vi "Main.vi"() -> ()   [LabVIEW 2018]
doc: "The myRIO Project template acquires acceleration data from the onboard accelerometer and displays the changes of acceleration values in a waveform chart."
uses:
  <vilib>/myRIO/Common/Instrument Driver Framework/myRIO v1.0/UART/vis/myRIO v1.0 Close UART.vi
  <vilib>/Utility/error.llb/Error Cluster From Error Code.vi
  <vilib>/myRIO/Common/Instrument Driver Framework/myRIO v1.0/PWM/vis/myRIO v1.0 Write PWM.vi
  <vilib>/myRIO/Common/Instrument Driver Framework/myRIO v1.0/AI/vis/myRIO v1.0 Read AI.vi
  <vilib>/myRIO/Common/Instrument Driver Framework/myRIO v1.0/DIO/vis/myRIO v1.0 Read DIO.vi
  <vilib>/myRIO/Common/Instrument Driver Framework/myRIO v1.0/DIO/vis/myRIO v1.0 Write DIO.vi
  <vilib>/myRIO/Common/Instrument Driver Framework/Utilities/vis/FPGA Ref Manager.vi
  <vilib>/myRIO/Common/Instrument Driver Framework/myRIO v1.0/myRIO v1.0 Reset FPGA.vi
  <vilib>/myRIO/Common/Instrument Driver Framework/myRIO v1.0/IRQ/vis/myRIO v1.0 IRQ Info FGV.vi
  <vilib>/myRIO/Common/Instrument Driver Framework/myRIO v1.0/IRQ/vis/myRIO v1.0 Timer IRQ Info FGV.vi
  <vilib>/myRIO/Common/Instrument Driver Framework/myRIO v1.0/IRQ/vis/myRIO v1.0 ISR Agent.vi
  <vilib>/myRIO/Instrument Drivers/Utilities/Utilities.lvlib
  <vilib>/myRIO/Instrument Drivers/Onboard IO/PWM/PWM.lvlib
  <vilib>/myRIO/Instrument Drivers/Onboard IO/AI/AI.lvlib
  <vilib>/myRIO/Instrument Drivers/Onboard IO/DIO/DIO.lvlib
panel:
  in  "Stepper frekvens":dbl=350.0
  out "ALL BOTTOM":bool
  out "ALL TOP":bool
  in  "Test bor (T = Amperestyring)":bool
  in  "DIR":bool
  in  "Endstops":bool
  in  "Manuel stepper?":bool
  in  "Enum":T1(ring)
  out "Batteri tilbage (%)":dbl
  out "Mean 50":dbl format="%0.2f"
  out "Mean 100":dbl format="%0.2f"
  in  "Threshold forskel":dbl=0.02 format="%#_13g"
  out "Duty Cycle":dbl
  in  "Styr manuelt?":bool=TRUE
  out "Waveform Chart":dbl(graph)
  out "Målt ampere":dbl
  in  "Bor - Frequency [Hz]":dbl=200.0
  in  "Bor - Duty Cycle":dbl=50.0
  out "error out":errorcluster
  in  "Stop":bool
  # "WIRING:\nBrun = GND\nOrange = PWM (A/DIO8)"
  # "STYRING AF SYSTEM!"
  # "100 = max\n50 = 0\n0 = -max"
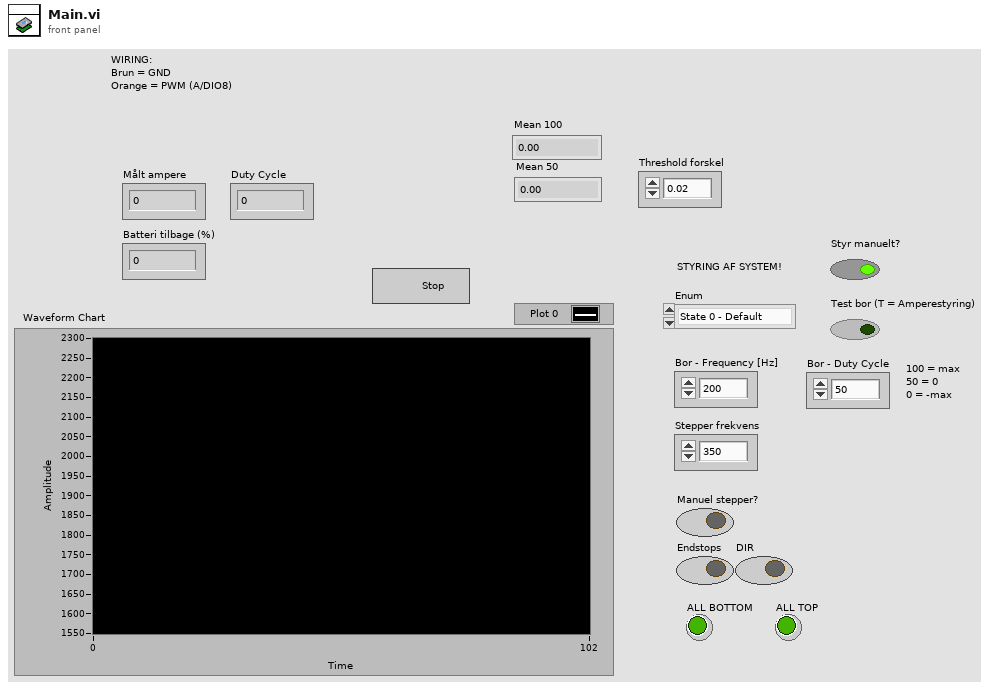
[diagram p1: front panel]
types:
  T1 = enum16{"State 0 - Default", "State 1 - Go down", "State 2 - Go up"}
  T2 = typedef "DIO.lvlib/DIO Reference.ctl" = cluster{"myRIO Reference":T3, "DIO Channels List":T7}
  T3 = typedef "myRIO Generic Hardware Reference.ctl" = cluster{"myRIO Model":T4, "myRIO Hardware Reference":T5}
  T4 = typedef "Hardware Version Enum.ctl" = enum16{"Unknown", "myRIO-1900", "myRIO-1950", "roboRIO", "NI ELVIS RIO CM", "ELVIS III"}
  T5 = typedef "myRIO v1.0 Reference.ctl" = cluster{"Generic FPGA Reference":T6, "Allow multiple opens":bool}
  T6 = typedef "Generic FPGA Reference.ctl" = refnum<k20>
  T7 = typedef "DIO Channels List.ctl" = T8[]
  T8 = typedef "DIO Channels Enum.ctl" = enum16{"Not Connected", "C/DIO0", "C/DIO1", "C/DIO2", "C/DIO3", "C/DIO4", "C/DIO5", "C/DIO6", "C/DIO7", "A/DIO0", "A/DIO1", "A/DIO2", "A/DIO3", "A/DIO4", "A/DIO5", "A/DIO6", "A/DIO7", "A/DIO8", "A/DIO9", "A/DIO10", "A/DIO11", "A/DIO12", "A/DIO13", "A/DIO14", "A/DIO15", "A/DIO16", "A/DIO17", "A/DIO18", "A/DIO19", "B/DIO0", "B/DIO1", "B/DIO2", "B/DIO3", "B/DIO4", "B/DIO5", "B/DIO6", "B/DIO7", "B/DIO8", "B/DIO9", "B/DIO10", "B/DIO11", "B/DIO12", "B/DIO13", "B/DIO14", "B/DIO15", "B/DIO16", "B/DIO17", "B/DIO18", "B/DIO19", "LED0", "LED1", "LED2", "LED3", "Button0", "DIO/DIO0", "DIO/DIO1", "DIO/DIO2", "DIO/DIO3", "DIO/DIO4", "DIO/DIO5", "DIO/DIO6", "DIO/DIO7", "DIO/DIO8", "DIO/DIO9", "SPI/CS0", "SPI/CS1", "SPI/CS2", "SPI/CS3", "LED RADIO (Green)", "LED RADIO (Red)", "LED COMM (Green)", "LED COMM (Red)", "LED MODE (Green)", "LED MODE (Red)"}
  T9 = typedef "PWM.lvlib/PWM Reference.ctl" = cluster{"myRIO Reference":T3, "PWM Channels Enum":T10, "PWM Configuration":T11}
  T10 = typedef "PWM Channels Enum.ctl" = enum16{"Not Connected", "C/PWM0", "C/PWM1", "A/PWM0", "A/PWM1", "A/PWM2", "A/PWM3", "A/PWM4", "A/PWM5", "A/PWM6", "A/PWM7", "A/PWM8", "A/PWM9", "A/PWM10", "A/PWM11", "A/PWM12", "A/PWM13", "A/PWM14", "A/PWM15", "A/PWM16", "A/PWM17", "A/PWM18", "A/PWM19", "B/PWM0", "B/PWM1", "B/PWM2", "B/PWM3", "B/PWM4", "B/PWM5", "B/PWM6", "B/PWM7", "B/PWM8", "B/PWM9", "B/PWM10", "B/PWM11", "B/PWM12", "B/PWM13", "B/PWM14", "B/PWM15", "B/PWM16", "B/PWM17", "B/PWM18", "B/PWM19", "PWM/PWM0", "PWM/PWM1", "PWM/PWM2", "PWM/PWM3", "PWM/PWM4", "PWM/PWM5", "PWM/PWM6", "PWM/PWM7", "PWM/PWM8", "PWM/PWM9"}
  T11 = typedef "PWM.lvlib/PWM Configuration.ctl" = cluster{"Frequency":dbl, "Duty Cycle":dbl}
  T12 = typedef "Accelerometer.lvlib/Accelerometer Reference.ctl" = cluster{"myRIO Reference":T3, "Accelerometer Channels List":T13, "LSB Weight":dbl}
  T13 = typedef "Accelerometer Channels List.ctl" = T14[]
  T14 = typedef "Accelerometer Channels Enum.ctl" = enum16{"Not Connected", "X-Axis", "Y-Axis", "Z-Axis"}
  T15 = typedef "AI.lvlib/AI Reference.ctl" = cluster{"myRIO Reference":T3, "AI Channels List":T16, "AI Scaling Constants List":T18}
  T16 = typedef "AI Channels List.ctl" = T17[]
  T17 = typedef "AI Channels Enum.ctl" = enum16{"Not Connected", "AudioIn/Left", "AudioIn/Right", "C/AI0", "C/AI1", "A/AI0", "A/AI1", "A/AI2", "A/AI3", "A/AI4", "A/AI5", "A/AI6", "A/AI7", "B/AI0", "B/AI1", "B/AI2", "B/AI3", "B/AI4", "B/AI5", "B/AI6", "B/AI7", "AI/AI0", "AI/AI1", "AI/AI2", "AI/AI3", "A/AI0 (DIFF)", "A/AI1 (DIFF)", "A/AI2 (DIFF)", "A/AI3 (DIFF)", "B/AI0 (DIFF)", "B/AI1 (DIFF)", "B/AI2 (DIFF)", "B/AI3 (DIFF)"}
  T18 = typedef "Analog Scaling Constants List.ctl" = T19[]
  T19 = typedef "Analog Scaling Constants.ctl" = cluster{"LSB Weight (Volts)":dbl, "Offset (Volts)":dbl, "Signed?":bool}
  T20 = typedef "SPI.lvlib/SPI Reference.ctl" = cluster{"myRIO Reference":T3, "SPI Channels Enum":T21, "SPI Configuration":T22}
  T21 = typedef "SPI Channels Enum.ctl" = enum16{"Not Connected", "A/SPI", "B/SPI", "SPI/SPI"}
  T22 = typedef "SPI.lvlib/SPI Configuration.ctl" = cluster{"Frequency [Hz]":dbl, "Clock Phase":T23, "Clock Polarity":T24, "Data Direction":T25, "Frame Length":T26}
  T23 = typedef "SPI Clock Phase.ctl" = enum8{"Leading", "Trailing"}
  T24 = typedef "SPI Clock Polarity.ctl" = enum8{"Low", "High"}
  T25 = typedef "SPI Data Direction.ctl" = enum8{"Most significant bit first", "Least significant bit first"}
  T26 = typedef "SPI Frame Length.ctl" = u8
  T27 = cluster{"B/DIO0 - Stepper Direction":T2, "B/DIO1 - Stepper1 Enable":T2, "B/DIO2 - Stepper2 Enable":T2, "B/DIO3 - Stepper3 Enable":T2, "B/DIO4 - Endstop Stepper1 Top":T2, "B/DIO11 - Endstop Stepper1 Bund":T2, "B/DIO12 - Endstop Stepper2 Top":T2, "B/DIO13 - Endstop Stepper2 Bund":T2, "B/DIO14 - Endstop Stepper3 Top":T2, "B/DIO15 - Endstop Stepper3 Bund":T2, "A/DIO0 - Cooler":T2, "A/DIO1 - Beacon drop (dio1)":T2, "A/DIO2 - Beacon drop (dio0)":T2, "A/DIO3 - QuickRelease (dio1)":T2, "A/DIO4 - QuickRelease (dio0)":T2, "A/DIO11 - LiDAR SPI CS":T2, "B/PWM0 - Stepper":T9, "B/PWM1 - Drill":T9, "A/PWM0 - Servo_Roll":T9, "A/PWM1 - Servo_Yaw":T9, "Acc. X-axis":T12, "Acc. Y-axis":T12, "B/AI0 - Drone Grounded F3":T15, "B/AI1 - Drone Drill Gear F4":T15, "B/AI2 - Beacon Drop F5":T15, "B/AI3 - Drone Drill Boost F6":T15, "A/AI0 - Drone Stepper F8":T15, "A/AI1 - Beacon Wiper":T15, "A/AI2 - QuickRelease Wiper":T15, "A/AI3 - Drill Current":T15, "A/SPI - LiDAR":T20, "B/UART - XBee":refnum<visa-resource-name>, "A/UART - A3 GPS":refnum<visa-resource-name>, "RIO Flashing LEDs":T2}
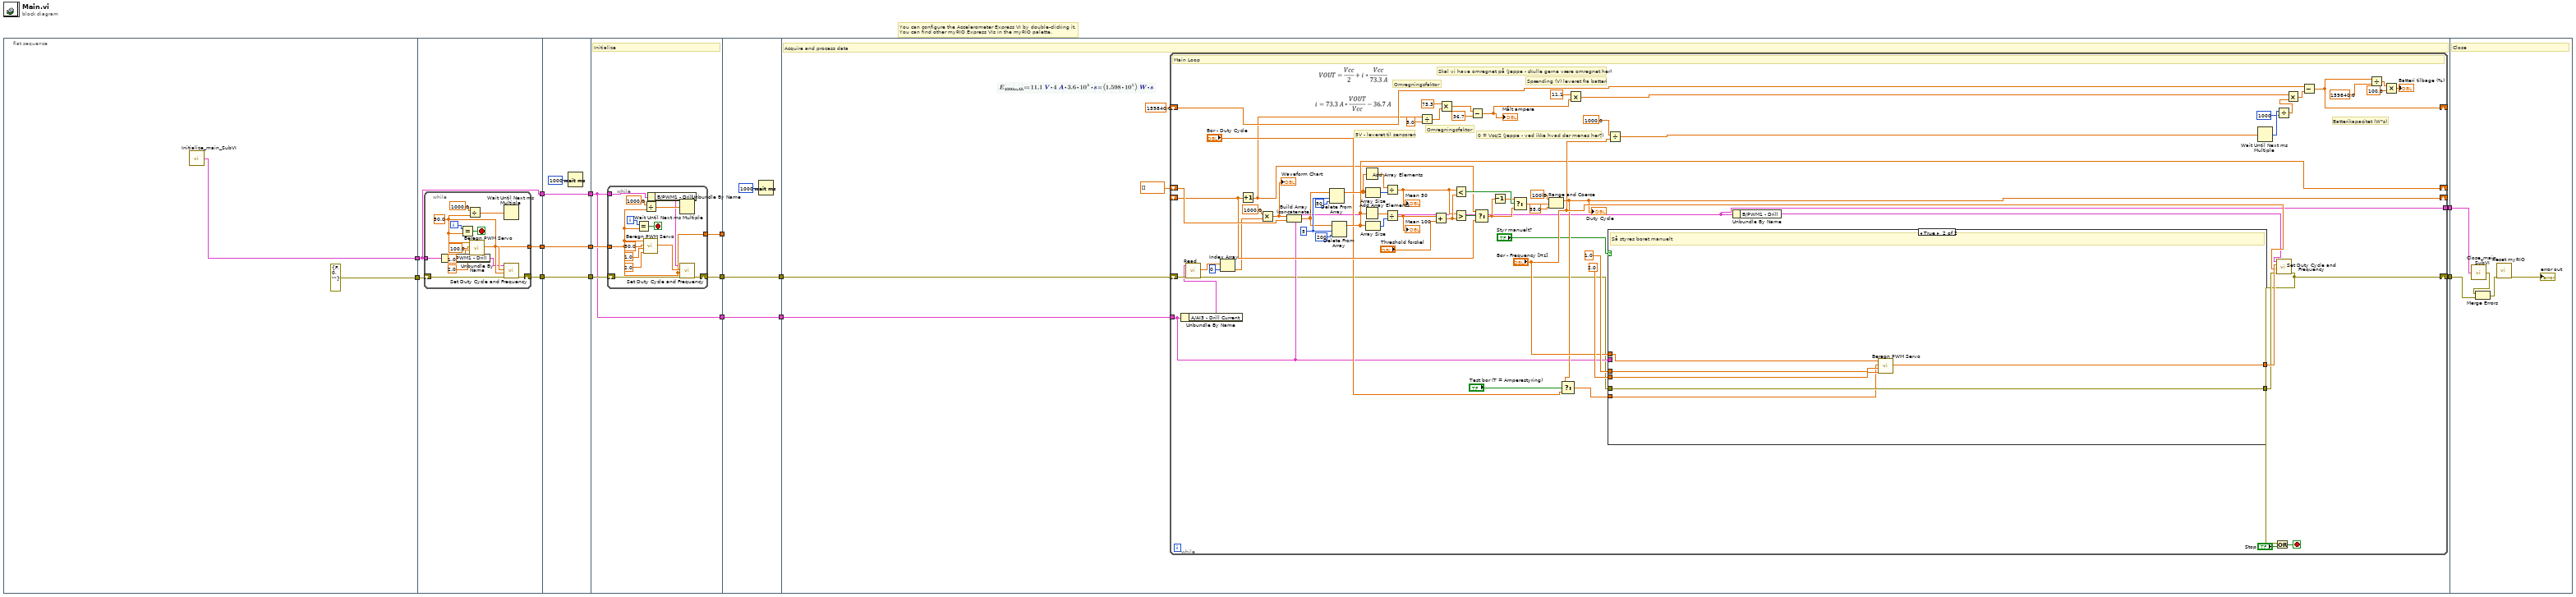
[diagram p0: block diagram]
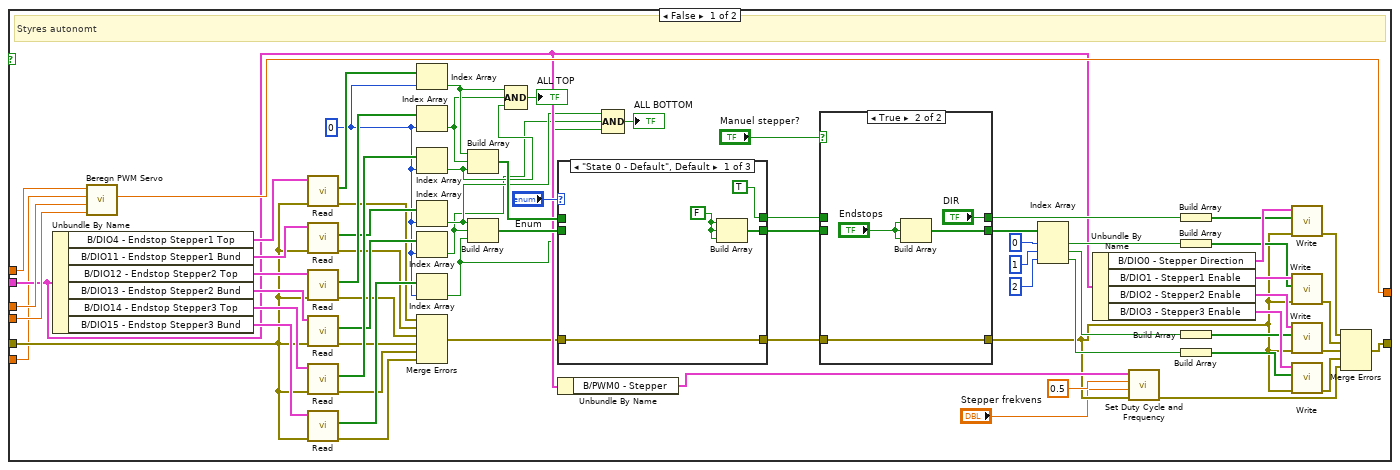
[diagram p2: hidden frame]
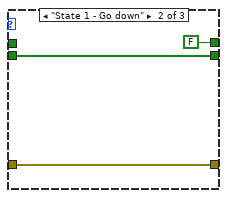
[diagram p4: hidden frame]
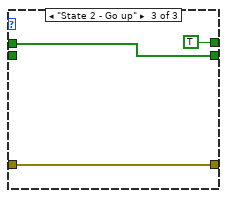
[diagram p5: hidden frame]
diagram:
  # "You can configure the Accelerometer Express VI by double-clicking it.\nYou can find other myRIO Express VIs in the myRIO palette."
  n1 = flat-sequence {
    tunnel: [w17] -> w8
    tunnel: [errorcluster {"status"=FALSE, "code"=0, "source"=""} ("error constant")] -> w2
    tunnel: [w21] -> w13
    tunnel: [w20] -> w11
    tunnel: w8 -> [w19]
    tunnel: [w19] -> w7
    tunnel: w2 -> [w18]
    tunnel: [w37] -> w14
    tunnel: w13 -> [w37]
    tunnel: [w36] -> w12
    tunnel: w11 -> [w36]
    tunnel: w7 -> [w35]
    tunnel: [w35] -> w6
    tunnel: w14 -> [w43]
    tunnel: w12 -> [w42]
    tunnel: [w40] -> w10
    tunnel: [w41] -> w9
    tunnel: w6 -> [w39]
    tunnel: [w39] -> w4
    tunnel: w10 -> [w57]
    tunnel: w9 -> [_]
    tunnel: [w58] -> w5
    tunnel: w4 -> [w58]
    tunnel: [w57] -> w3
    tunnel: [w65] -> w15
    tunnel: w5 -> [w62]
    tunnel: w3 -> [w61]
    tunnel: [w60] -> w1
    tunnel: w15 -> [w226]
    tunnel: w1 -> [w224]
    frame #0 {
      n2 = call "Initialize_main_SubVI.vi"() -> ("output cluster"=w17:T27)
    }
    frame #1 {
      n3 = while {
        tunnel: [w26] -> w21
        shift-right: [w29] -> w20
        shift-left: w18 -> [w30]
        tunnel: w19 -> [w23]
        i -> [w28]
        stop <- w24 stop-if-true
        w26 = 50.0 ("Frequency [Hz]")
        n4 = Unbundle By Name(w23) -> ("B/PWM1 - Drill"=w22:T9)
        n5 = Equal?(x=w28, y=w26) -> (x = y?=w24:bool)
        n6 = Divide(x=1000.0, y=w26) -> (x/y=w27:dbl)
        n7 = call "Beregn PWM Servo.vi"("Max (ms puls bredde)"=2.0, "Min (ms puls bredde)"=1.0, "Duty Cycle"=100.0, "Frekvens"=w26) -> ("Output Dutycycle til PWM Servo"=w31:dbl)  [unwired: 7 in]
        n8 = Wait Until Next ms Multiple(millisecond multiple=w27) -> ()  [unwired: 1 out]
        n9 = call <vilib>:"Set Duty Cycle and Frequency.vi"("error in (no error)"=w30, "Frequency [Hz]"=w26, "Duty Cycle"=w31, "PWM Ref In"=w22) -> ("error out"=w29:errorcluster)  [unwired: 5 in, 1 out]
      }
    }
    frame #2 {
      n10 = Wait (ms)(milliseconds to wait=u32 1000) -> ()  [unwired: 1 out]
    }
    frame #3 {
      # "Initialize"
      n11 = while {
        tunnel: [w46] -> w41
        shift-right: [w51] -> w40
        shift-left: w42 -> [w52]
        tunnel: w43 -> [w46]
        tunnel: w39 -> [w45]
        i -> [w50]
        stop <- w47 stop-if-true
        n12 = Equal?(x=w50, y=w46) -> (x = y?=w47:bool)
        n13 = call "Beregn PWM Servo.vi"("Max (ms puls bredde)"=2.0, "Min (ms puls bredde)"=1.0, "Duty Cycle"=50.0, "Frekvens"=w46) -> ("Output Dutycycle til PWM Servo"=w53:dbl)  [unwired: 7 in]
        n14 = Divide(x=1000.0, y=w46) -> (x/y=w49:dbl)
        n15 = Unbundle By Name(w45) -> ("B/PWM1 - Drill"=w44:T9)
        n16 = Wait Until Next ms Multiple(millisecond multiple=w49) -> ()  [unwired: 1 out]
        n17 = call <vilib>:"Set Duty Cycle and Frequency.vi"("error in (no error)"=w52, "Frequency [Hz]"=w46, "Duty Cycle"=w53, "PWM Ref In"=w44) -> ("error out"=w51:errorcluster)  [unwired: 5 in, 1 out]
      }
    }
    frame #4 {
      n18 = Wait (ms)(milliseconds to wait=u32 1000) -> ()  [unwired: 1 out]
    }
    frame #5 {
      # "Acquire and process data"
      n19 = while {
        shift-right: [w69] -> w65
        shift-left: w61 -> [w118]
        shift-right: [w104] -> _
        shift-left: dbl[] [] -> [w128]
        shift-right: [w77] -> _
        shift-left: _ -> [w125]
        shift-right: [w82] -> _
        shift-left: 159840.0 -> [w83]
        tunnel: w62 -> [w72]
        tunnel: [w72] -> w60
        stop <- w131 stop-if-true
        w111 = 5 ("length")
        # "Batterikapacitet (W*s)"
        # "Spænding (V) leveret fra batteri"
        # "Omregningsfaktor"
        # "Omregningsfaktor"
        # "5V - leveret til sensoren"
        # "Skal vi have omregnet på (Jeppe - skulle gerne være omregnet her)"
        # "0 = Vcc/2 (Jeppe - ved ikke hvad der menes her?)"
        # "Main Loop"
        n20 = Unbundle By Name(w72) -> ("A/AI3 - Drill Current"=w74:T15)
        n21 = call <vilib>:"Read.vi"("error in (no error)"=w118, "AI Ref In"=w74) -> ("error out"=w71:errorcluster, "Values"=w117:dbl[])  [unwired: 7 in, 1 out]
        n22 = Index Array(array=w117, index=0) -> (element=w98:dbl)
        n23 = Increment(x=w125) -> (x+1=w68:dbl)
        n24 = Multiply(x=1000.0, y=w98) -> (x*y=w96:dbl)
        "Waveform Chart" <- w96
        n25 = Build Array (concatenate)(w96, w128) -> (w109:dbl[])
        n26 = Delete From Array(array=w109, length=w111, index=50) -> (array with subset deleted=w100:dbl[])  [unwired: 1 out]
        n27 = Delete From Array(array=w109, length=w111, index=200) -> (array with subset deleted=w104:dbl[])  [unwired: 1 out]
        n28 = Add Array Elements(numeric array=w100) -> (sum=w101:dbl)
        n29 = Add Array Elements(numeric array=w104) -> (sum=w106:dbl)
        n30 = Array Size(array=w100) -> (size(s)=w102:i32)
        n31 = Array Size(array=w104) -> (size(s)=w105:i32)
        n32 = Divide(x=w101, y=w102) -> (x/y=w99:dbl)
        "Mean 50" <- w99
        n33 = Divide(x=w106, y=w105) -> (x/y=w103:dbl)
        "Mean 100" <- w103
        n34 = Divide(x=w68, y=5.0) -> (x/y=w94:dbl)
        n35 = Add(x=w103, y="Threshold forskel") -> (x+y=w108:dbl)
        n36 = Multiply(x=73.3, y=w94) -> (x*y=w92:dbl)
        n37 = Less?(x=w99, y=w108) -> (x < y?=w124:bool)
        n38 = Greater?(x=w99, y=w108) -> (0:w126:bool)
        n39 = Subtract(x=w92, y=36.7) -> (x-y=w89:dbl)
        "Målt ampere" <- w89
        n40 = Select(t=w68, s=w126, f=w125) -> (s? t:f=w123:dbl)
        n41 = Decrement(x=w123) -> (x-1=w122:dbl)
        n42 = Select(t=w122, s=w124, f=w123) -> (s? t:f=w121:dbl)
        n43 = In Range and Coerce(upper limit=100.0, x=w121, lower limit=55.0) -> (coerced(x)=w77:dbl)  [unwired: 1 out]
        "Duty Cycle" <- w77
        n44 = Select(t=w77, s="Test bor (T = Amperestyring)", f="Bor - Duty Cycle") -> (s? t:f=w66:dbl)
        n45 = Multiply(x=11.1, y=w89) -> (x*y=w88:dbl)
        n46 = Divide(x=1000.0, y="Bor - Frequency [Hz]") -> (x/y=w114:dbl)
        n47 = case shown="True" "Styr manuelt?" {
          tunnel: 2.0 ("Max (ms puls bredde)") -> [w200 w223]
          tunnel: 1.0 ("Min (ms puls bredde)") -> [w198 w222]
          tunnel: [w197 w221] -> w116
          tunnel: "Bor - Frequency [Hz]" -> [w199 w220]
          tunnel: w72 -> [w161 _]
          tunnel: w71 -> [w158 w219]
          tunnel: [w143 w219] -> w70
          tunnel: w66 -> [w133 w218]
          frame False {
            w182 = 0 ("index")
            # "Styres autonomt"
            n48 = Unbundle By Name(w161) -> ("B/DIO4 - Endstop Stepper1 Top"=w194:T2, "B/DIO11 - Endstop Stepper1 Bund"=w193:T2, "B/DIO12 - Endstop Stepper2 Top"=w192:T2, "B/DIO13 - Endstop Stepper2 Bund"=w191:T2, "B/DIO14 - Endstop Stepper3 Top"=w190:T2, "B/DIO15 - Endstop Stepper3 Bund"=w189:T2)
            n49 = call "Beregn PWM Servo.vi"("Max (ms puls bredde)"=w200, "Min (ms puls bredde)"=w198, "Duty Cycle"=w133, "Frekvens"=w199) -> ("Output Dutycycle til PWM Servo"=w197:dbl)  [unwired: 7 in]
            n50 = call <vilib>:"Read.vi"("error in (no error)"=w158, "DIO Ref In"=w194) -> ("error out"=w157:errorcluster, "Values"=w183:bool[])  [unwired: 7 in, 1 out]
            n51 = call <vilib>:"Read.vi"("error in (no error)"=w158, "DIO Ref In"=w193) -> ("error out"=w156:errorcluster, "Values"=w184:bool[])  [unwired: 7 in, 1 out]
            n52 = call <vilib>:"Read.vi"("error in (no error)"=w158, "DIO Ref In"=w192) -> ("error out"=w155:errorcluster, "Values"=w185:bool[])  [unwired: 7 in, 1 out]
            n53 = call <vilib>:"Read.vi"("error in (no error)"=w158, "DIO Ref In"=w191) -> ("error out"=w154:errorcluster, "Values"=w186:bool[])  [unwired: 7 in, 1 out]
            n54 = call <vilib>:"Read.vi"("error in (no error)"=w158, "DIO Ref In"=w190) -> ("error out"=w153:errorcluster, "Values"=w187:bool[])  [unwired: 7 in, 1 out]
            n55 = call <vilib>:"Read.vi"("error in (no error)"=w158, "DIO Ref In"=w189) -> ("error out"=w152:errorcluster, "Values"=w188:bool[])  [unwired: 7 in, 1 out]
            n56 = Index Array(array=w183, index=w182) -> (element=w142:bool)
            n57 = Index Array(array=w185, index=w182) -> (element=w141:bool)
            n58 = Index Array(array=w187, index=w182) -> (element=w140:bool)
            n59 = Index Array(array=w184, index=w182) -> (element=w137:bool)
            n60 = Index Array(array=w186, index=w182) -> (element=w136:bool)
            n61 = Index Array(array=w188, index=w182) -> (element=w135:bool)
            n62 = Merge Errors(w157, w156, w155, w154, w153, w152) -> (w151:errorcluster)
            n63 = Build Array(w142, w141, w140) -> (w180:bool[])
            n64 = Build Array(w137, w136, w135) -> (w181:bool[])
            n65 = Compound Arithmetic op=AND(w142, w141, w140) -> (→"ALL TOP":bool)
            n66 = case shown="\"State 0 - Default\", Default" "Enum" {
              tunnel: [w209 w214 w217] -> w165
              tunnel: w181 -> [_ w214 _]
              tunnel: w180 -> [_ _ w217]
              tunnel: [TRUE FALSE TRUE] -> w163
              tunnel: w151 -> [w208 w212 w215]
              tunnel: [w208 w212 w215] -> w150
              frame "State 0 - Default", Default {
                w210 = FALSE
                n67 = Build Array(w210, w210, w210) -> (w209:bool[])
              }
              frame "State 1 - Go down" {
              }
              frame "State 2 - Go up" {
              }
            }
            n68 = Unbundle By Name(w161) -> ("B/PWM0 - Stepper"=w160:T9)
            n69 = Compound Arithmetic op=AND(w137, w136, w135) -> (→"ALL BOTTOM":bool)
            n70 = case shown="True" "Manuel stepper?" {
              tunnel: w165 -> [w203 _]
              tunnel: [w203 w207] -> w164
              tunnel: w163 -> [w202 _]
              tunnel: [w202 "DIR"] -> w162
              tunnel: w150 -> [w201 w204]
              tunnel: [w201 w204] -> w149
              frame False {
              }
              frame True {
                n71 = Build Array("Endstops", "Endstops", "Endstops") -> (w207:bool[])
              }
            }
            n72 = Index Array(array=w164, index #1=0 ("index"), index #2=1 ("index"), index #3=2 ("index")) -> (element #1=w172:bool, element #2=w170:bool, element #3=w168:bool)
            n73 = Unbundle By Name(w161) -> ("B/DIO0 - Stepper Direction"=w195:T2, "B/DIO1 - Stepper1 Enable"=w178:T2, "B/DIO2 - Stepper2 Enable"=w177:T2, "B/DIO3 - Stepper3 Enable"=w176:T2)
            n74 = call <vilib>:"Set Duty Cycle and Frequency.vi"("error in (no error)"=w149, "Frequency [Hz]"="Stepper frekvens", "Duty Cycle"=0.5, "PWM Ref In"=w160) -> ("error out"=w144:errorcluster)  [unwired: 5 in, 1 out]
            n75 = Build Array(w162) -> (w179:bool[])
            n76 = Build Array(w172) -> (w171:bool[])
            n77 = Build Array(w170) -> (w169:bool[])
            n78 = Build Array(w168) -> (w167:bool[])
            n79 = call <vilib>:"Write.vi"("error in (no error)"=w149, "Values"=w179, "DIO Ref In"=w195) -> ("error out"=w148:errorcluster)  [unwired: 6 in, 1 out]
            n80 = call <vilib>:"Write.vi"("error in (no error)"=w149, "Values"=w171, "DIO Ref In"=w178) -> ("error out"=w147:errorcluster)  [unwired: 6 in, 1 out]
            n81 = call <vilib>:"Write.vi"("error in (no error)"=w149, "Values"=w169, "DIO Ref In"=w177) -> ("error out"=w146:errorcluster)  [unwired: 6 in, 1 out]
            n82 = call <vilib>:"Write.vi"("error in (no error)"=w149, "Values"=w167, "DIO Ref In"=w176) -> ("error out"=w145:errorcluster)  [unwired: 6 in, 1 out]
            n83 = Merge Errors(w148, w147, w146, w145, w144) -> (w143:errorcluster)
          }
          frame True {
            # "Så styres boret manuelt"
            n84 = call "Beregn PWM Servo.vi"("Max (ms puls bredde)"=w223, "Min (ms puls bredde)"=w222, "Duty Cycle"=w218, "Frekvens"=w220) -> ("Output Dutycycle til PWM Servo"=w221:dbl)  [unwired: 7 in]
          }
        }
        n85 = Unbundle By Name(w72) -> ("B/PWM1 - Drill"=w73:T9)
        n86 = Wait Until Next ms Multiple(millisecond multiple=w114) -> (millisecond timer value=w87:u32)
        n87 = Divide(x=w87, y=u32 1000) -> (x/y=w85:dbl)
        n88 = call <vilib>:"Set Duty Cycle and Frequency.vi"("error in (no error)"=w70, "Frequency [Hz]"="Bor - Frequency [Hz]", "Duty Cycle"=w116, "PWM Ref In"=w73) -> ("error out"=w69:errorcluster)  [unwired: 5 in, 1 out]
        n89 = Or(x=w69, y="Stop") -> (x .or. y?=w131:bool)
        n90 = Multiply(x=w88, y=w85) -> (x*y=w84:dbl)
        n91 = Subtract(x=w83, y=w84) -> (x-y=w82:dbl)
        n92 = Divide(x=w82, y=159840.0) -> (x/y=w80:dbl)
        n93 = Multiply(x=w80, y=100.0) -> (x*y=→"Batteri tilbage (%)":dbl)
      }
    }
    frame #6 {
      # "Close"
      n94 = call "Close_main_SubVI.vi"("output cluster"=w224) -> ("error constant"=w227:errorcluster)
      n95 = Merge Errors(w227, w226) -> (w225:errorcluster)
      n96 = call <vilib>:"Reset myRIO.vi"("error in (no error)"=w225) -> ("error out"=→"error out":errorcluster)  [unwired: 10 in]
    }
  }
